vi "Close.vi"(8 "error in (no error)":errorcluster {"code" format="Error %.0f"}, 11 "VIDoc Printer - Confluence In":refnum<class "VIDoc Printer - Confluence.lvclass">) -> (0 "error out":errorcluster {"code" format="Error %.0f"})   [LabVIEW 2023, in "VIDoc Printer - Confluence.lvlib" / "VIDoc Printer - Confluence.lvclass"]
uses:
  VIDoc Printer - Confluence.lvclass
  VIDoc Printer - Confluence.lvclass/VIDoc Printer - Confluence.ctl
  Printer/VIDoc Printer.lvclass
  <userlib>/_PetranWay/LabVIEW Confluence API/Source/Confluence/Confluence Connection/Confluence.lvclass
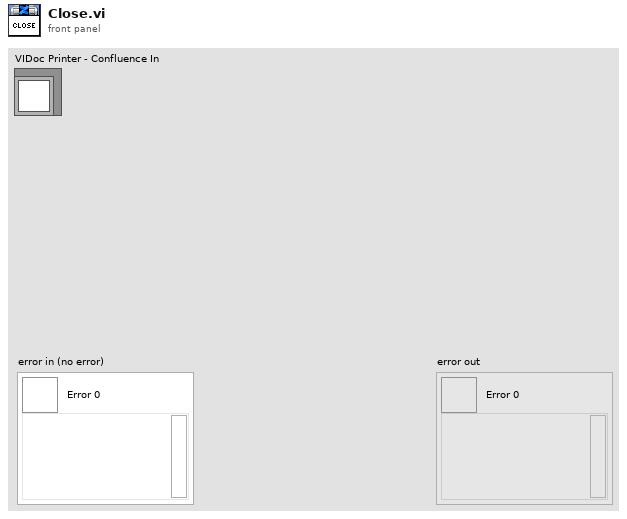
[diagram p1: front panel]
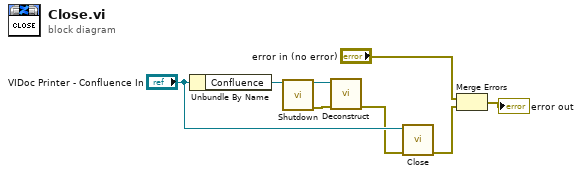
[diagram p0: block diagram]
diagram:
  n1 = Unbundle By Name("VIDoc Printer - Confluence In") -> ("Confluence"=w4:refnum<class "Confluence.lvclass">)
  n2 = call-dynamic "Shutdown.vi"("Confluence in"=w4) -> ("Confluence out"=w7:refnum<class "Confluence.lvclass">, "error out"=w6:errorcluster)  [unwired: 13 in]
  n3 = call-dynamic "Deconstruct.vi"("error in (no error)"=w6, "Confluence in"=w7) -> ("error out"=w1:errorcluster)  [unwired: 9 in]
  n4 = call-parent "Close.vi"("error in (no error)"=w1, "VIDoc Printer In"="VIDoc Printer - Confluence In") -> ("error out"=w8:errorcluster)  [unwired: 9 in]
  n5 = Merge Errors("error in (no error)", w8) -> (→"error out":errorcluster)
